vi "WS1021 demo Main.vi"   [LabVIEW 2020]
panel:
  # "Digitally Tunable Capacitor"
types:
  T1 = enum32{"Invalid", "Standard", "Closed", "Hidden", "Minimized", "Maximized"}
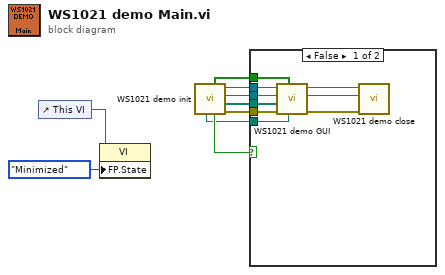
[diagram p0: block diagram]
diagram:
  n1 = control-ref of="This VI"() -> (w3:refnum<vi>)
  n2 = property class="VI"(reference=w3, "FP.State"=T1."Minimized" ("Front Panel Window:State")) -> ()  [unwired: 1 in, 2 out]
  n3 = call "WS1021 demo init.vi"() -> ("Error Out"=w9:errorcluster, "De-embedding files"=w6:path[], "Toggle 8.lvclass"=w7:refnum<class "Toggle 8.lvclass">, "Vector Network Analyzer.lvclass"=w8:refnum<class "Vector Network Analyzer.lvclass">, "Cancelled"=w5:bool, "VNA ports out"=w4:bool[], "Error Limits 2"=w1:path)  [unwired: 5 in]
  n4 = case shown="False" w5 {
    tunnel: w9 -> [w18 _]
    tunnel: w8 -> [w17 _]
    tunnel: w7 -> [w14 _]
    tunnel: w6 -> [w12 _]
    tunnel: w4 -> [w11 _]
    tunnel: w1 -> [w10 _]
    frame False {
      n5 = call "WS1021 demo GUI.vi"("Error Limits file"=w10, "VNA ports"=w11, "Error In"=w18, "De-embedding files"=w12, "Toggle 8.lvclass"=w14, "Vector Network Analyzer.lvclass"=w17) -> ("Error Out"=w16:errorcluster, "Toggle 8.lvclass 2"=w13:refnum<class "Toggle 8.lvclass">, "Vector Network Analyzer.lvclass 2"=w15:refnum<class "Vector Network Analyzer.lvclass">)  [unwired: 3 in]
      n6 = call "WS1021 demo close.vi"("Error In"=w16, "Toggle 8.lvclass"=w13, "Vector Network Analyzer.lvclass"=w15) -> ()  [unwired: 8 in, 1 out]
    }
    frame True {
    }
  }
